vi "Write Message Tag.vi"(8 "error in (no error)":errorcluster, 10 "Message Tag":string, 11 "abs_EventLog in":refnum<class "abs_EventLog.lvclass">) -> (0 "error out":errorcluster, 3 "abs_EventLog out":refnum<class "abs_EventLog.lvclass">)   [LabVIEW 2021, in "abs_EventLog.lvclass"]
uses:
  abs_EventLog.lvclass
  abs_EventLog.lvclass/abs_EventLog.ctl
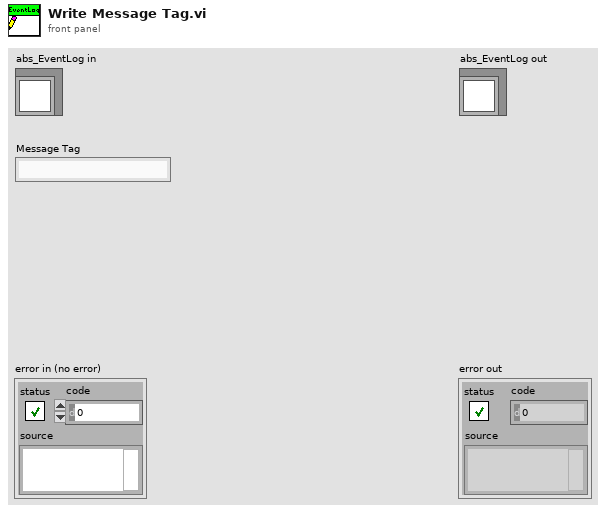
[diagram p1: front panel]
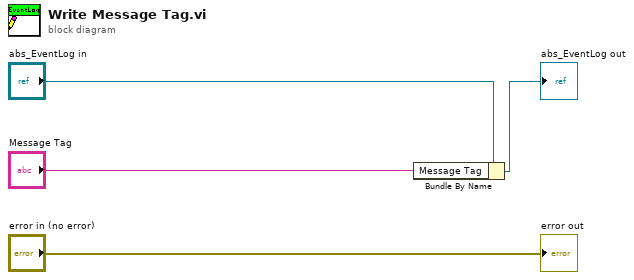
[diagram p0: block diagram]
diagram:
  n1 = Bundle By Name(cluster="abs_EventLog in", "Message Tag"="Message Tag") -> (→"abs_EventLog out":refnum<class "abs_EventLog.lvclass">)
  "error out" <- "error in (no error)"
